vi "Motors_Encoders_Sensors.vi"(0 "Motor 4 speed":dbl(slide) scale=-100.0..100.0, 1 "Motor 3 speed":dbl(slide) scale=-100.0..100.0, 2 "Reset Encoder 1":bool, 3 "Reset Encoder in":bool, 4 "Reset Encoder 3":bool, 6 "Motor 2 speed":dbl(slide) scale=-100.0..100.0, 7 "Reset Encoder 4":bool, 8 "Motor 1 speed":dbl(slide) scale=-100.0..100.0, 9 "Koffset [cm]":dbl, 11 "Kscale [cm-V]":dbl=27.5) -> (10 "IR Range":dbl, 12 "Vo [V]":dbl format="%.2f", 13 "Counter 4":i32, 14 "Counter 1":i32, 15 "Ping Distance (m) 1":dbl, 16 "Counter 2":i32, 17 "Ping Distance (m) 2":dbl, 18 "Counter 3":i32, 19 "error out":errorcluster)   [LabVIEW 2018]
uses:
  <vilib>/myRIO/Instrument Drivers/Onboard IO/DIO/typedefs/DIO Reference.ctl
  <vilib>/myRIO/Common/Instrument Driver Framework/Utilities/typedefs/myRIO Generic Hardware Reference.ctl
  <vilib>/myRIO/Common/Instrument Driver Framework/Utilities/typedefs/Hardware Version Enum.ctl
  <vilib>/myRIO/Common/Instrument Driver Framework/Utilities/typedefs/myRIO v1.0 Reference.ctl
  <vilib>/myRIO/Common/Instrument Driver Framework/Utilities/typedefs/Generic FPGA Reference.ctl
  <vilib>/myRIO/Common/Instrument Driver Framework/myRIO v1.0/DIO/typedefs/DIO Channels List.ctl
  <vilib>/myRIO/Common/Instrument Driver Framework/myRIO v1.0/DIO/typedefs/DIO Channels Enum.ctl
  <vilib>/userdefined/High Color/nirio_resource_hc.ctl
  <vilib>/myRIO/Instrument Drivers/Onboard IO/PWM/typedefs/PWM Reference.ctl
  <vilib>/myRIO/Common/Instrument Driver Framework/myRIO v1.0/PWM/typedefs/PWM Channels Enum.ctl
  <vilib>/myRIO/Instrument Drivers/Onboard IO/PWM/typedefs/PWM Configuration.ctl
  <vilib>/myRIO/Instrument Drivers/Onboard IO/AI/typedefs/AI Reference.ctl
  <vilib>/myRIO/Common/Instrument Driver Framework/myRIO v1.0/AI/typedefs/AI Channels List.ctl
  <vilib>/myRIO/Common/Instrument Driver Framework/myRIO v1.0/AI/typedefs/AI Channels Enum.ctl
  <vilib>/myRIO/Common/Instrument Driver Framework/Utilities/typedefs/Analog Scaling Constants List.ctl
  <vilib>/myRIO/Common/Instrument Driver Framework/Utilities/typedefs/Analog Scaling Constants.ctl
  <vilib>/myRIO/Common/Instrument Driver Framework/myRIO v1.0/Encoder/typedefs/Encoder Signal Mode.ctl
  <vilib>/myRIO/Instrument Drivers/Onboard IO/Encoder/typedefs/Encoder Reference.ctl
  <vilib>/myRIO/Common/Instrument Driver Framework/myRIO v1.0/Encoder/typedefs/Encoder Channels Enum.ctl
  <vilib>/myRIO/Common/Instrument Driver Framework/myRIO v1.0/Encoder/typedefs/Encoder Configuration v1.0.ctl
  <vilib>/myRIO/Common/Instrument Driver Framework/Utilities/vis/Is FPGA Ref Available.vi
  <vilib>/myRIO/Common/Instrument Driver Framework/myRIO v1.0/DIO/vis/myRIO v1.1 Open DIO.vi
  <vilib>/myRIO/Instrument Drivers/Onboard IO/DIO/vis/Write.vi
  <vilib>/myRIO/Common/Instrument Driver Framework/myRIO v1.0/PWM/vis/myRIO v1.1 Open PWM.vi
  <vilib>/myRIO/Instrument Drivers/Onboard IO/PWM/vis/Set Duty Cycle and Frequency.vi
  <vilib>/myRIO/Common/Instrument Driver Framework/myRIO v1.0/AI/vis/myRIO v1.1 Open AI.vi
  <vilib>/myRIO/Instrument Drivers/Onboard IO/AI/vis/Read.vi
  <vilib>/myRIO/Common/Instrument Driver Framework/myRIO v1.0/Encoder/vis/myRIO v1.1 Open Encoder.vi
  <vilib>/myRIO/Instrument Drivers/Onboard IO/Encoder/vis/Read.vi
  <vilib>/myRIO/Common/Instrument Driver Framework/Utilities/vis/Validate Channels.vi
  <vilib>/myRIO/Common/Instrument Driver Framework/myRIO v1.0/DIO/vis/myRIO v1.0 Reserve DIO.vi
  <vilib>/myRIO/Common/Instrument Driver Framework/myRIO v1.0/PWM/vis/myRIO v1.0 Reserve PWM.vi
  <vilib>/myRIO/Common/Instrument Driver Framework/myRIO v1.0/AI/vis/myRIO v1.0 Reserve AI.vi
  <vilib>/myRIO/Common/Instrument Driver Framework/myRIO v1.0/Encoder/vis/myRIO v1.0 Reserve Encoder.vi
  <vilib>/myRIO/Common/Instrument Driver Framework/myRIO v1.0/Resource Manager/vis/myRIO v1.0 Reserve Channel List.vi
  <vilib>/myRIO/Common/Instrument Driver Framework/myRIO v1.0/DIO/vis/myRIO v1.0 Build MUX Configuration DIO.vi
  <vilib>/myRIO/Common/Instrument Driver Framework/myRIO v1.0/PWM/vis/myRIO v1.0 Build MUX Configuration PWM.vi
  <vilib>/myRIO/Common/Instrument Driver Framework/myRIO v1.0/AI/vis/myRIO v1.0 Build MUX Configuration AI.vi
  <vilib>/myRIO/Common/Instrument Driver Framework/myRIO v1.0/Encoder/vis/myRIO v1.0 Build MUX Configuration Encoder.vi
  <vilib>/myRIO/Common/Instrument Driver Framework/myRIO v1.0/Resource Manager/vis/myRIO v1.0 Reserve Channel.vi
  <vilib>/myRIO/Common/Instrument Driver Framework/myRIO v1.0/Resource Manager/vis/myRIO v1.0 Unreserve Channel.vi
  <vilib>/myRIO/Common/Instrument Driver Framework/myRIO v1.0/Resource Manager/vis/myRIO v1.0 Create Configuration List.vi
  <vilib>/myRIO/Common/Instrument Driver Framework/myRIO v1.0/Resource Manager/vis/myRIO v1.0 Build Mutex Name.vi
  <vilib>/Utility/VariantDataType/GetNumericInfo.vi
  <vilib>/Utility/error.llb/Error Cluster From Error Code.vi
  <vilib>/myRIO/Common/Instrument Driver Framework/myRIO v1.0/myRIO v1.1 Open.vi
  <vilib>/myRIO/Common/Instrument Driver Framework/Utilities/vis/IO Manager.vi
  <vilib>/myRIO/Common/Instrument Driver Framework/Utilities/vis/Configuration Manager.vi
  <vilib>/myRIO/Common/Instrument Driver Framework/myRIO v1.0/Resource Manager/vis/myRIO v1.0 Configure IO.vi
  <vilib>/myRIO/Common/Instrument Driver Framework/myRIO v1.0/myRIO v1.0 Close.vi
  <vilib>/myRIO/Common/Instrument Driver Framework/myRIO v1.0/DIO/vis/myRIO v1.0 Write DIO.vi
  <vilib>/myRIO/Common/Instrument Driver Framework/myRIO v1.0/PWM/vis/myRIO v1.0 Write PWM.vi
  <vilib>/myRIO/Common/Instrument Driver Framework/myRIO v1.0/AI/vis/myRIO v1.0 Get Scaling Constants AI.vi
  <vilib>/myRIO/Common/Instrument Driver Framework/myRIO v1.0/AI/vis/myRIO v1.0 Read AI.vi
  <vilib>/myRIO/Common/Instrument Driver Framework/myRIO v1.0/Encoder/vis/myRIO v1.0 Configure Encoder.vi
  <vilib>/myRIO/Common/Instrument Driver Framework/myRIO v1.0/Encoder/vis/myRIO v1.0 Read Encoder.vi
  <vilib>/myRIO/Express VI/Onboard IO/DO/DO Express VI.xnode
  <vilib>/myRIO/Instrument Drivers/Onboard IO/DIO/vis/myRIO DIO Open.xnode
  <vilib>/myRIO/Express VI/Onboard IO/PWM/PWM Express VI.xnode
  <vilib>/myRIO/Instrument Drivers/Onboard IO/PWM/vis/myRIO PWM Open.xnode
  <vilib>/myRIO/Express VI/Onboard IO/AI/AI Express VI.xnode
  <vilib>/myRIO/Instrument Drivers/Onboard IO/AI/vis/myRIO AI Open.xnode
  <vilib>/myRIO/Express VI/Onboard IO/Encoder/Encoder Express VI.xnode
  <vilib>/myRIO/Instrument Drivers/Onboard IO/Encoder/vis/myRIO Encoder Open.xnode
  <vilib>/myRIO/Common/Instrument Driver Framework/myRIO v1.0/Encoder/typedefs/Encoder Count Direction Enum.ctl
  <vilib>/myRIO/Instrument Drivers/Onboard IO/Encoder/Encoder.lvlib
  <vilib>/ptbypt/NI_PtbyPt.lvlib
  <vilib>/myRIO/Instrument Drivers/Onboard IO/AI/AI.lvlib
  <vilib>/myRIO/Instrument Drivers/Onboard IO/DIO/DIO.lvlib
  <vilib>/myRIO/Instrument Drivers/Onboard IO/PWM/PWM.lvlib
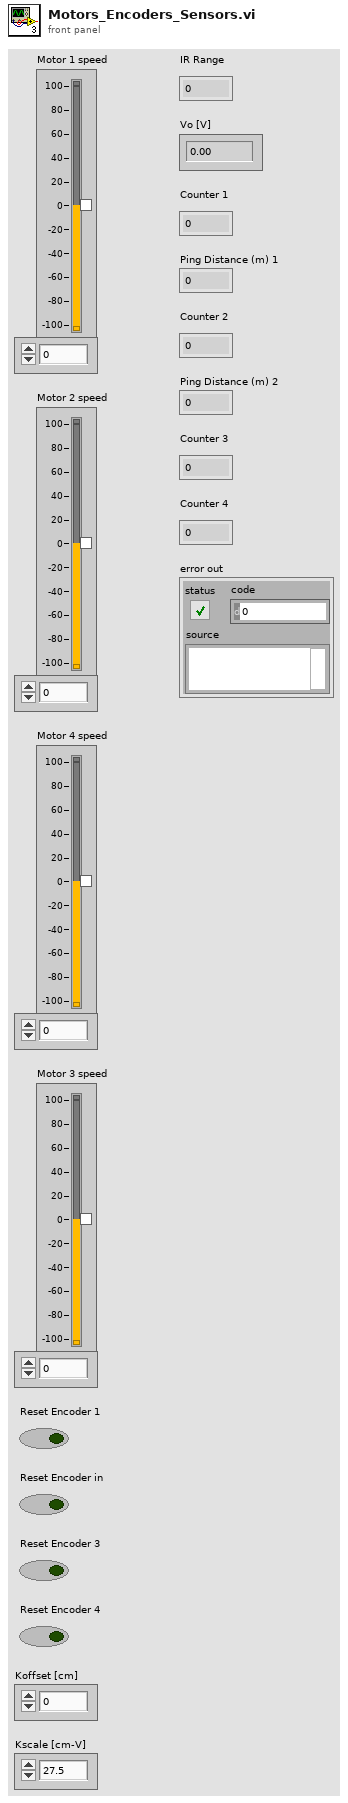
[diagram p1: front panel]
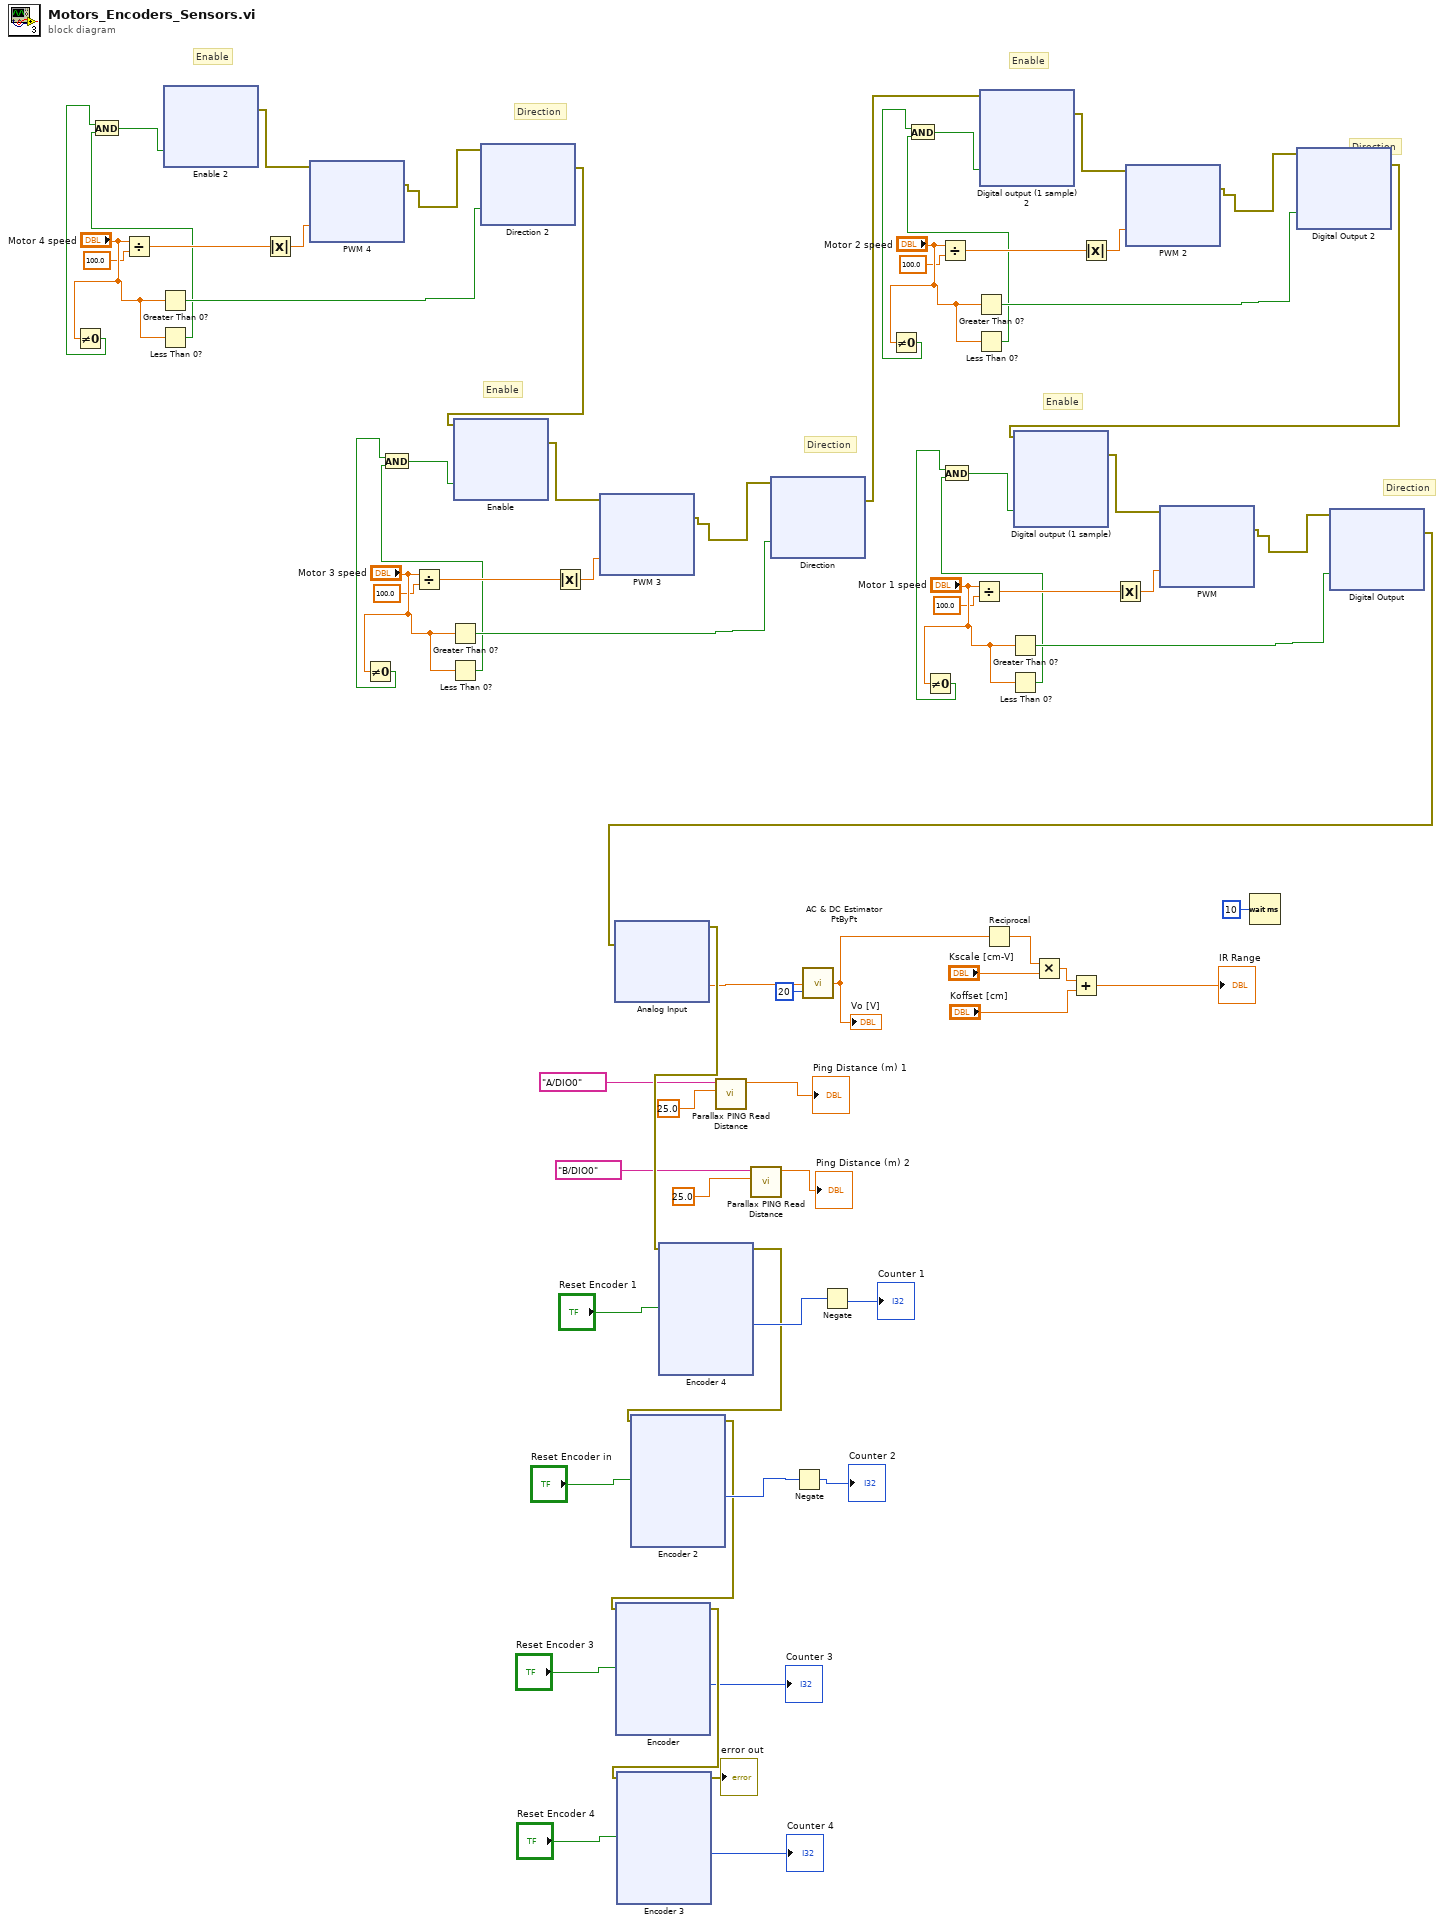
[diagram p0: block diagram]
diagram:
  # "Enable"
  # "Direction"
  # "Enable"
  # "Direction"
  # "Enable"
  # "Direction"
  # "Enable"
  # "Direction"
  n1 = Not Equal To 0?(x="Motor 4 speed") -> (x != 0?=w64:bool)
  n2 = Divide(x="Motor 4 speed", y=100.0) -> (x/y=w65:dbl)
  n3 = Greater Than 0?(x="Motor 4 speed") -> (x > 0?=w68:bool)
  n4 = Less Than 0?(x="Motor 4 speed") -> (x < 0?=w62:bool)
  n5 = And(x=w64, y=w62) -> (x .and. y?=w69:bool)
  n6 = xnode "Enable 2"("B/DIO7 (Pin 25)"=w69) -> ("error out"=w61:errorcluster)  [unwired: 1 in]
  n7 = Absolute Value(x=w65) -> (abs(x)=w66:dbl)
  n8 = xnode "PWM 4"("Duty Cycle"=w66, "error in (no error)"=w61) -> ("error out"=w60:errorcluster)
  n9 = Not Equal To 0?(x="Motor 3 speed") -> (x != 0?=w52:bool)
  n10 = Divide(x="Motor 3 speed", y=100.0) -> (x/y=w53:dbl)
  n11 = Greater Than 0?(x="Motor 3 speed") -> (x > 0?=w57:bool)
  n12 = Less Than 0?(x="Motor 3 speed") -> (x < 0?=w50:bool)
  n13 = And(x=w52, y=w50) -> (x .and. y?=w58:bool)
  n14 = xnode "Direction 2"("B/DIO13 (Pin 26)"=w68, "error in (no error)"=w60) -> ("error out"=w67:errorcluster)
  n15 = xnode "Enable"("A/DIO7 (Pin 25)"=w58, "error in (no error)"=w67) -> ("error out"=w49:errorcluster)
  n16 = Absolute Value(x=w53) -> (abs(x)=w54:dbl)
  n17 = xnode "PWM 3"("Duty Cycle"=w54, "error in (no error)"=w49) -> ("error out"=w48:errorcluster)
  n18 = call "Parallax PING Read Distance.vi"("Temperature (deg C)"=25.0, "myRIO DIO Channel"=tag "A/DIO0") -> ("Distance (m)"=→"Ping Distance (m) 1":dbl)  [unwired: 8 in, 1 out]
  n19 = call "Parallax PING Read Distance.vi"("Temperature (deg C)"=25.0, "myRIO DIO Channel"=tag "B/DIO0") -> ("Distance (m)"=→"Ping Distance (m) 2":dbl)  [unwired: 8 in, 1 out]
  n20 = xnode "Direction"("A/DIO13 (Pin 26)"=w57, "error in (no error)"=w48) -> ("error out"=w55:errorcluster)
  n21 = Not Equal To 0?(x="Motor 2 speed") -> (x != 0?=w42:bool)
  n22 = Not Equal To 0?(x="Motor 1 speed") -> (x != 0?=w32:bool)
  n23 = Divide(x="Motor 2 speed", y=100.0) -> (x/y=w43:dbl)
  n24 = Divide(x="Motor 1 speed", y=100.0) -> (x/y=w35:dbl)
  n25 = Greater Than 0?(x="Motor 2 speed") -> (x > 0?=w45:bool)
  n26 = Less Than 0?(x="Motor 2 speed") -> (x < 0?=w40:bool)
  n27 = And(x=w42, y=w40) -> (x .and. y?=w46:bool)
  n28 = xnode "Digital output (1 sample) 2"("B/DIO5 (Pin 21)"=w46, "error in (no error)"=w55) -> ("error out"=w39:errorcluster)
  n29 = Greater Than 0?(x="Motor 1 speed") -> (x > 0?=w33:bool)
  n30 = Less Than 0?(x="Motor 1 speed") -> (x < 0?=w30:bool)
  n31 = And(x=w32, y=w30) -> (x .and. y?=w34:bool)
  n32 = Absolute Value(x=w43) -> (abs(x)=w44:dbl)
  n33 = Absolute Value(x=w35) -> (abs(x)=w36:dbl)
  n34 = xnode "PWM 2"("Duty Cycle"=w44, "error in (no error)"=w39) -> ("error out"=w38:errorcluster)
  n35 = Wait (ms)(milliseconds to wait=u32 10) -> ()  [unwired: 1 out]
  n36 = xnode "Digital Output 2"("B/DIO6 (Pin 23)"=w45, "error in (no error)"=w38) -> ("error out"=w56:errorcluster)
  n37 = xnode "Digital output (1 sample)"("A/DIO5 (Pin 21)"=w34, "error in (no error)"=w56) -> ("error out"=w29:errorcluster)
  n38 = xnode "PWM"("Duty Cycle"=w36, "error in (no error)"=w29) -> ("error out"=w28:errorcluster)
  n39 = xnode "Digital Output"("A/DIO6 (Pin 23)"=w33, "error in (no error)"=w28) -> ("error out"=w70:errorcluster)
  n40 = xnode "Analog Input"("error in (no error)"=w70) -> ("A/AI0 (Pin 3)"=w15:dbl, "error out"=w22:errorcluster)
  n41 = xnode "Encoder 4"("Reset Counter"="Reset Encoder 1", "error in (no error)"=w22) -> ("Counter Value"=w74:i32, "error out"=w23:errorcluster)  [unwired: 2 out]
  n42 = xnode "Encoder 2"("Reset Counter"="Reset Encoder in", "error in (no error)"=w23) -> ("Counter Value"=w72:i32, "error out"=w24:errorcluster)  [unwired: 2 out]
  n43 = xnode "Encoder"("Reset Counter"="Reset Encoder 3", "error in (no error)"=w24) -> ("Counter Value"=→"Counter 3":i32, "error out"=w25:errorcluster)  [unwired: 2 out]
  n44 = xnode "Encoder 3"("Reset Counter"="Reset Encoder 4", "error in (no error)"=w25) -> ("Counter Value"=→"Counter 4":i32, "error out"=→"error out":errorcluster)  [unwired: 2 out]
  n45 = Negate(x=w72) -> (-x=→"Counter 2":i32)
  n46 = call <vilib>:"AC & DC Estimator PtByPt.vi"("signal"=w15, "sample length"=20) -> ("DC estimate (V)"=w16:dbl)  [unwired: 1 in, 2 out]
  "Vo [V]" <- w16
  n47 = Negate(x=w74) -> (-x=→"Counter 1":i32)
  n48 = Reciprocal(x=w16) -> (1/x=w13:dbl)
  n49 = Multiply(x=w13, y="Kscale [cm-V]") -> (x*y=w19:dbl)
  n50 = Add(x=w19, y="Koffset [cm]") -> (x+y=→"IR Range":dbl)
